vi "Config Ramp.vi"(0 "VISA resource name":refnum<visa-resource-name>, 7 "Rate Value (0.001)":dbl=0.001 min=0.001 max=10.0 step=0.001 format="%.3f", 9 "Ramping On/Off (F: Ramping Off)":bool, 11 "error in (no error)":errorcluster) -> (4 "VISA resource name out":refnum<visa-resource-name>, 15 "error out":errorcluster)   [LabVIEW 2024, in "Lake Shore Cryotronics 370.lvlib"]
doc: "This VI configures the parameters of setpoint ramp."
uses:
  Lake Shore Cryotronics 370.lvlib
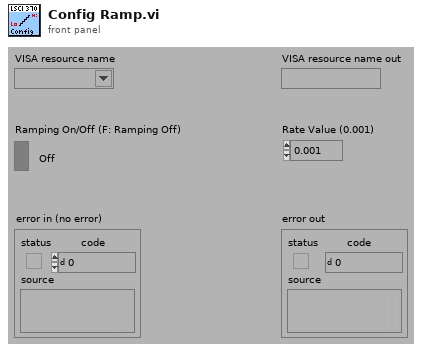
[diagram p1: front panel]
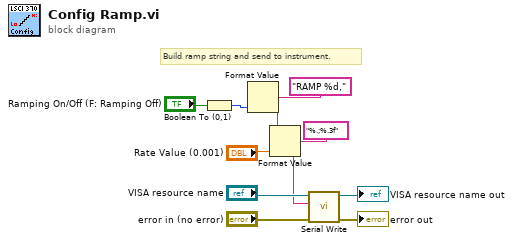
[diagram p0: block diagram]
diagram:
  # "Build ramp string and send to instrument."
  n1 = Boolean To (0,1)(Boolean="Ramping On/Off (F: Ramping Off)") -> (0, 1=w10:i16)
  n2 = Format Value(format string="RAMP %d,", value (0)=w10) -> (output string=w6:string)  [unwired: 1 in]
  n3 = Format Value(string ("")=w6, format string="%.;%.3f", value (0)="Rate Value (0.001)") -> (output string=w1:string)
  n4 = call "Serial Write.vi"("error in (no error)"="error in (no error)", "Write Buffer (\"\")"=w1, "VISA resource name"="VISA resource name") -> ("error out"=→"error out":errorcluster, "VISA resource name out"=→"VISA resource name out":refnum<visa-resource-name>)  [unwired: 6 in, 1 out]
